vi "적외선 센서.vi"() -> ()   [LabVIEW 2018]
panel:
  out "측정거리":dbl
  in  "stop (F)":bool caption="정지(F)"
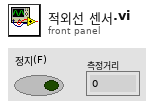
[diagram p1: front panel]
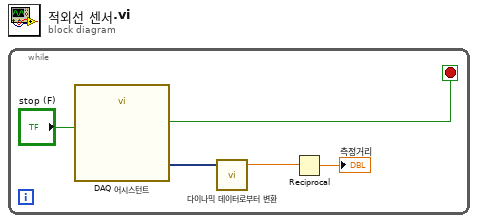
[diagram p0: block diagram]
diagram:
  n1 = while {
    stop <- w4 stop-if-true
    n2 = call "DAQ 어시스턴트"("stop (F)"="stop (F)") -> ("data"=w3:dynamicdata, "stopped"=w4:bool)  [unwired: 15 in, 2 out]
    n3 = call "다이나믹 데이터로부터 변환"("Dynamic Data Type"=w3) -> ("Scalar"=w2:dbl)  [unwired: 3 in]
    n4 = Reciprocal(x=w2) -> (1/x=→"측정거리":dbl)
  }
